vi "DX3003DS.vi"(4 "Current(mA)":dbl, 6 "Voltage(V)":dbl, 8 "error in":errorcluster caption="错误输入（无错误）", 9 "ON/Off":bool, 10 "Mode":T1(ring), 11 "MyIndex":u8) -> (0 "error out":errorcluster caption="错误输出", 1 "CurOut(mA)":u16, 2 "VoltOut":dbl, 3 "OK?":bool)   [LabVIEW 2015]
uses:
  <vilib>/Instr/_visa.llb/VISA Configure Serial Port (Instr).vi
panel:
  out "VISA":refnum<visa-resource-name>
  out "读取缓冲区":string
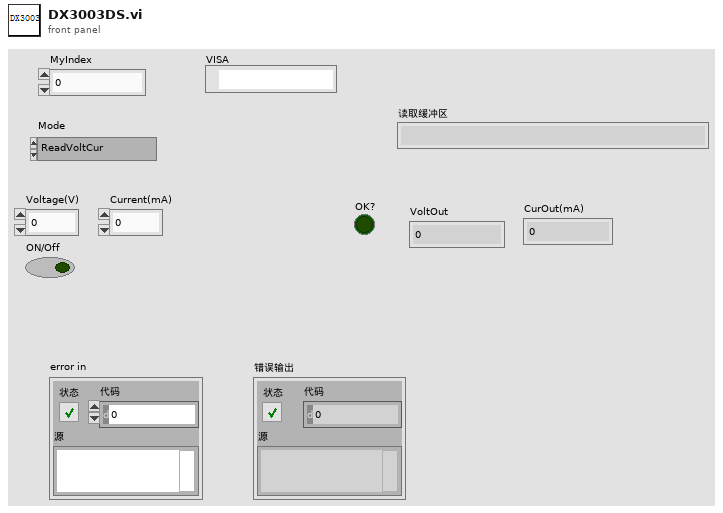
[diagram p1: front panel]
types:
  T1 = enum16{"ReadVoltCur", "SetVolCur", "ON/OFF", "SetVoltage", "SetCurrent"}
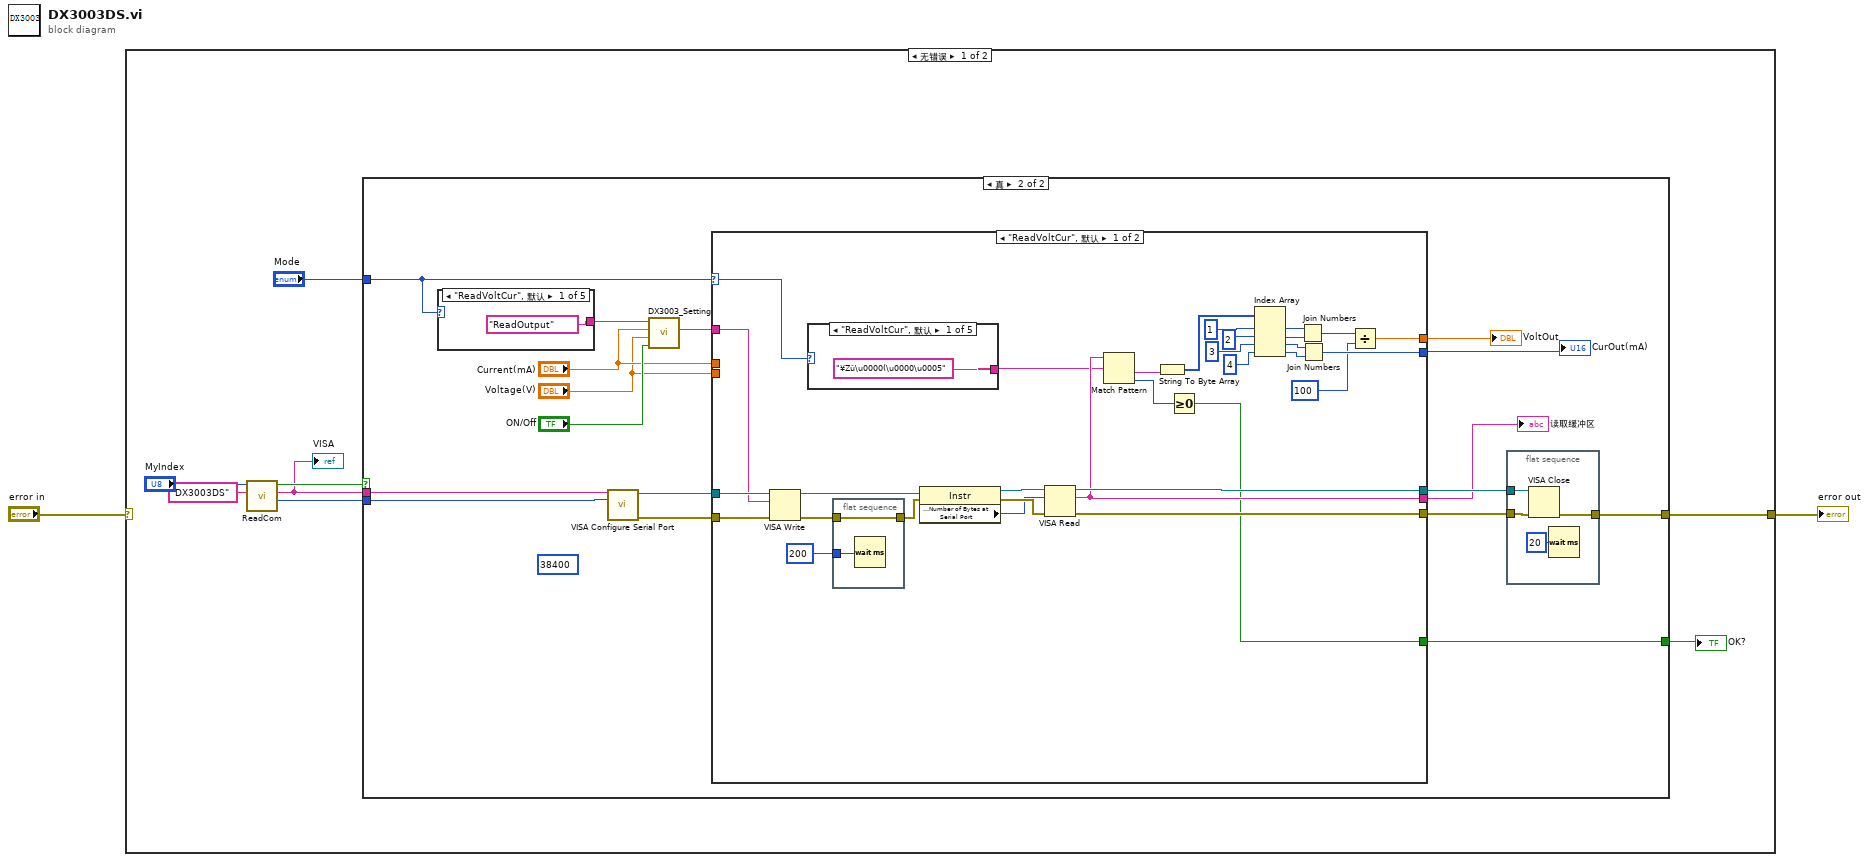
[diagram p0: block diagram]
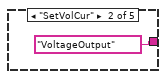
[diagram p3: hidden frame]
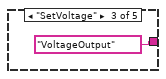
[diagram p4: hidden frame]
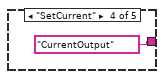
[diagram p5: hidden frame]
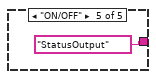
[diagram p6: hidden frame]
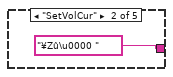
[diagram p7: hidden frame]
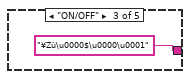
[diagram p8: hidden frame]
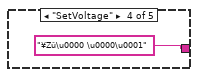
[diagram p9: hidden frame]
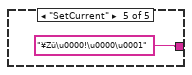
[diagram p10: hidden frame]
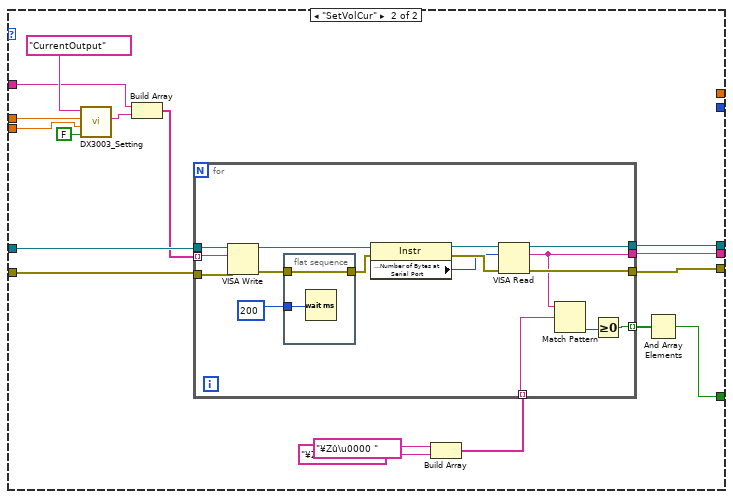
[diagram p11: hidden frame]
diagram:
  n1 = case shown="无错误" "error in" {
    selector: "error in" -> [_ w110]
    tunnel: [w3 w110] -> w1
    frame No Error {
      n2 = call "ReadCom.vi"("仪器名称"="DX3003DS", "MyIndex"="MyIndex") -> ("Baudrate"=w4:i32, "COM"=w6:string, "OK?"=w7:bool)  [unwired: 7 in]
      "VISA" <- w6
      n3 = case shown="真" w7 {
        tunnel: [_ w17] -> w10
        tunnel: w6 -> [_ w14]
        tunnel: "Mode" -> [_ w13]
        tunnel: w4 -> [_ w12]
        tunnel: [_ w11] -> w3
        frame False {
        }
        frame True {
          (unwired) u32 38400 ("baud rate (9600)")
          n4 = case shown="\"ReadVoltCur\", 默认" w13 {
            tunnel: ["ReadOutput" ("Setup") "VoltageOutput" ("Setup") "VoltageOutput" ("Setup") "CurrentOutput" ("Setup") "StatusOutput" ("Setup")] -> w22
            frame "ReadVoltCur", Default {
            }
            frame "SetVolCur" {
            }
            frame "SetVoltage" {
            }
            frame "SetCurrent" {
            }
            frame "ON/OFF" {
            }
          }
          n5 = call-poly "VISA Configure Serial Port"("VISA resource name"=w14, "baud rate (9600)"=w12) -> ("VISA resource name out"=w27:refnum<visa-resource-name>, "error out"=w25:errorcluster)  [unwired: 12 in]
          n6 = call "DX3003_Setting.vi"("ON/Off"="ON/Off", "Voltage(V)"="Voltage(V)", "Current(mA)"="Current(mA)", "Setup"=w22) -> ("Command"=w20:string)  [unwired: 7 in]
          n7 = case shown="\"ReadVoltCur\", 默认" w13 {
            selector: w13 -> [w51 _]
            tunnel: w27 -> [w63 w87]
            tunnel: [w60 w86] -> w26
            tunnel: w25 -> [w59 w85]
            tunnel: [w57 w84] -> w24
            tunnel: [w50 w83] -> w23
            tunnel: w20 -> [w52 w77]
            tunnel: "Current(mA)" -> [_ w82]
            tunnel: "Voltage(V)" -> [_ w79]
            tunnel: [w47 w71] -> w17
            tunnel: [w33 _] -> w16
            tunnel: [w36 _] -> w15
            frame "ReadVoltCur", Default {
              n8 = VISA Write(VISA resource name=w63, write buffer=w52, error in (no error)=w59) -> (VISA resource name out=w62:refnum<visa-resource-name>, error out=w56:errorcluster)  [unwired: 1 out]
              n9 = case shown="\"ReadVoltCur\", 默认" w51 {
                tunnel: ["¥Zû\u0000(\u0000\u0005" "¥Zû\u0000 " "¥Zû\u0000$\u0000\u0001" "¥Zû\u0000 \u0000\u0001" "¥Zû\u0000!\u0000\u0001"] -> w49
                frame "ReadVoltCur", Default {
                }
                frame "SetVolCur" {
                }
                frame "ON/OFF" {
                }
                frame "SetVoltage" {
                }
                frame "SetCurrent" {
                }
              }
              n10 = flat-sequence {
                tunnel: w56 -> [w69]
                tunnel: u32 200 ("等待时间（毫秒）") -> [w70]
                tunnel: [w69] -> w53
                frame #0 {
                  n11 = Wait (ms)(milliseconds to wait=w70) -> ()  [unwired: 1 out]
                }
              }
              n12 = property class="Instr"(reference=w62, error in=w53) -> (reference out=w61:refnum<visa-resource-name>, error out=w58:errorcluster, "Serial Settings:Number of Bytes at Serial Port"=w55:u32)
              n13 = VISA Read(VISA resource name=w61, byte count=w55, error in (no error)=w58) -> (VISA resource name out=w60:refnum<visa-resource-name>, read buffer=w50:string, error out=w57:errorcluster)  [unwired: 1 out]
              n14 = Match Pattern(string=w50, regular expression=w49) -> (after substring=w46:string, offset past match=w48:i32)  [unwired: 1 in, 2 out]
              n15 = String To Byte Array(string=w46) -> (unsigned byte array=w45:u8[])
              n16 = Greater Or Equal To 0?(x=w48) -> (x >= 0?=w47:bool)
              n17 = Index Array(array=w45, index #1=1 ("索引"), index #2=2 ("索引"), index #3=3 ("索引"), index #4=4 ("索引")) -> (element #1=w40:u8, element #2=w39:u8, element #3=w38:u8, element #4=w37:u8)
              n18 = Join Numbers(hi=w40, lo=w39) -> ((hi.lo)=w35:u16)
              n19 = Join Numbers(hi=w38, lo=w37) -> ((hi.lo)=w36:u16)
              n20 = Divide(x=w35, y=u16 100) -> (x/y=w33:dbl)
            }
            frame "SetVolCur" {
              n21 = call "DX3003_Setting.vi"("ON/Off"=FALSE, "Voltage(V)"=w79, "Current(mA)"=w82, "Setup"="CurrentOutput") -> ("Command"=w78:string)  [unwired: 7 in]
              n22 = Build Array(w77, w78) -> (w76:string[])
              n23 = Build Array("¥Zû\u0000 ", "¥Zû\u0000!") -> (w73:string[])
              n24 = for {
                tunnel: [w91] -> w83
                tunnel: w76 -> [w92] mode=indexing
                tunnel: w73 -> [w90] mode=indexing
                tunnel: [w88] -> w72 mode=indexing
                tunnel: w85 -> [w99]
                tunnel: [w97] -> w84
                tunnel: w87 -> [w103]
                tunnel: [w100] -> w86
                n25 = VISA Write(VISA resource name=w103, write buffer=w92, error in (no error)=w99) -> (VISA resource name out=w102:refnum<visa-resource-name>, error out=w96:errorcluster)  [unwired: 1 out]
                n26 = flat-sequence {
                  tunnel: w96 -> [w104]
                  tunnel: u32 200 ("等待时间（毫秒）") -> [w105]
                  tunnel: [w104] -> w93
                  frame #0 {
                    n27 = Wait (ms)(milliseconds to wait=w105) -> ()  [unwired: 1 out]
                  }
                }
                n28 = property class="Instr"(reference=w102, error in=w93) -> (reference out=w101:refnum<visa-resource-name>, error out=w98:errorcluster, "Serial Settings:Number of Bytes at Serial Port"=w95:u32)
                n29 = VISA Read(VISA resource name=w101, byte count=w95, error in (no error)=w98) -> (VISA resource name out=w100:refnum<visa-resource-name>, read buffer=w91:string, error out=w97:errorcluster)  [unwired: 1 out]
                n30 = Match Pattern(string=w91, regular expression=w90) -> (offset past match=w89:i32)  [unwired: 1 in, 3 out]
                n31 = Greater Or Equal To 0?(x=w89) -> (x >= 0?=w88:bool)
              }
              n32 = And Array Elements(Boolean array=w72) -> (logical AND=w71:bool)
            }
          }
          "读取缓冲区" <- w23
          "VoltOut" <- w16
          "CurOut(mA)" <- w15
          n33 = flat-sequence {
            tunnel: w26 -> [w109]
            tunnel: w24 -> [w108]
            tunnel: [w106] -> w11
            frame #0 {
              n34 = VISA Close(VISA resource name=w109, error in (no error)=w108) -> (error out=w106:errorcluster)
              n35 = Wait (ms)(milliseconds to wait=u32 20 ("等待时间（毫秒）")) -> ()  [unwired: 1 out]
            }
          }
        }
      }
      "OK?" <- w10
    }
    frame Error {
    }
  }
  "error out" <- w1
